vi "VNA_Easy_Loop_Sweep_CenterFreq.vi"(4 "CentreF Start (Hz)":dbl=1000000000.0 format="%#_8p", 5 "Transport":refnum<class "Transport.lvclass">, 7 "VNA Address":refnum<visa-resource-name>="GPIB0::15::INSTR", 9 "sweep type (0 : linear)":u16(ring) items=["linear sweep", "logarithmic sweep", "frequency list", "CW time sweep", "power sweep"], 10 "sweep time (sec)":dbl=1.0 format="%.2f", 11 "num points":u16(ring)=8 items=["3", "11", "21 ('20) / 26 ('53)", "51", "101", "201", "401", "801", "1601"]) -> (2 "Polar plot":cluster{dbl[], sgl[]}[](graph))   [LabVIEW 2020]
uses:
  <userlib>/LevyLab/Transport/Transport/Transport.lvclass
  <userlib>/LevyLab/Transport/Transport/Transport.lvclass/Transport.ctl
  <userlib>/LevyLab/Transport/Control Experiment/Control Experiment.lvclass/Control Experiment.ctl
  <userlib>/LevyLab/Transport/Control Experiment/Control Experiment.lvclass
  <userlib>/LevyLab/Instrument Framework/Instrument Types/Cryostat/Instrument.Cryostat.lvclass
  <instrlib>/Agilent 87XX Series/Agilent 87XX Series.lvlib
panel:
  in  "Power (dBm)":dbl=10.0
  in  "CentreF Step (Hz)":dbl=50000000.0 format="%#_8p"
  in  "CentreF End (Hz)":dbl=1200000000.0 format="%#_8p"
  out "Data 2":cluster{dbl[], dbl[]}[](graph)
  out "B Field (T)":dbl=-0.0001169
  out "Temperature (K)":dbl=300.0009
  in  "Vg (V)":dbl
  in  "Ids (mA)":dbl=9.5
  in  "Vds (V)":dbl=1.3
  in  "Experiment Description":string="D1 1/2\nT = 300K\nVdc1 =AO1 (100kohm shunt) = 0 V\nVcd2 = AO2  (100kohm shunt) = 0 V\nP_vna = 10 dBm \nCentreF = 1G to 1.2G\nSpan=50M"
  in  "Experiment Folder":string="06-100K_bias0V"
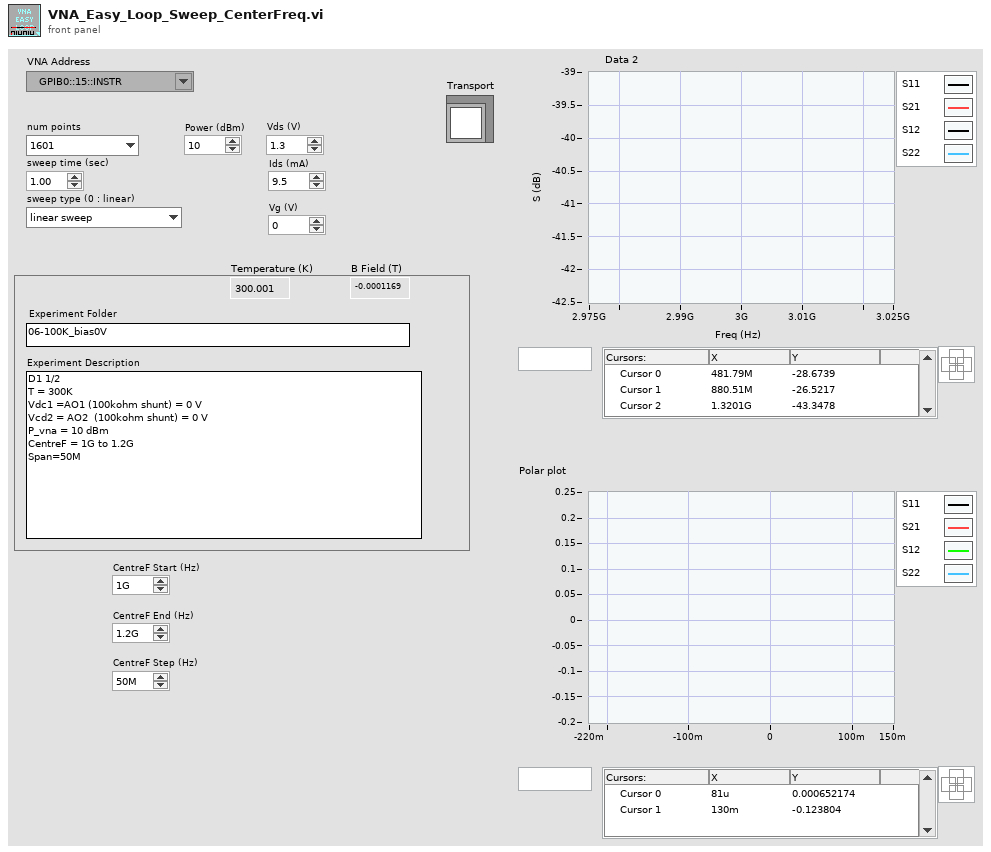
[diagram p1: front panel]
types:
  T1 = enum32{"Bad", "Idle", "Run top level", "Running"}
  T2 = typedef "Control Experiment.lvclass/Instrument Classes--cluster.ctl" = cluster{"DAQ":refnum<class "Instrument.LockinAPI.lvclass">, "Amplifier":refnum<class "Instrument.Amplifier.lvclass">, "Temperature":refnum<class "Instrument.Cryostat.lvclass">, "Magnet":refnum<class "Instrument.Cryostat.lvclass">, "Rotator":refnum<class "Instrument.Cryostat.lvclass">, "Level":refnum<class "Instrument.Cryostat.lvclass">, "Capacitance":refnum<class "Instrument.CBridge.lvclass">, "Delay Line":refnum<class "Instrument.DelayLine.lvclass">, "Strain Cell":refnum<class "Instrument.Strain.lvclass">, "VNA":refnum<class "Instrument.VNA.lvclass">, "Source":refnum<class "Instrument.VSource.lvclass">}
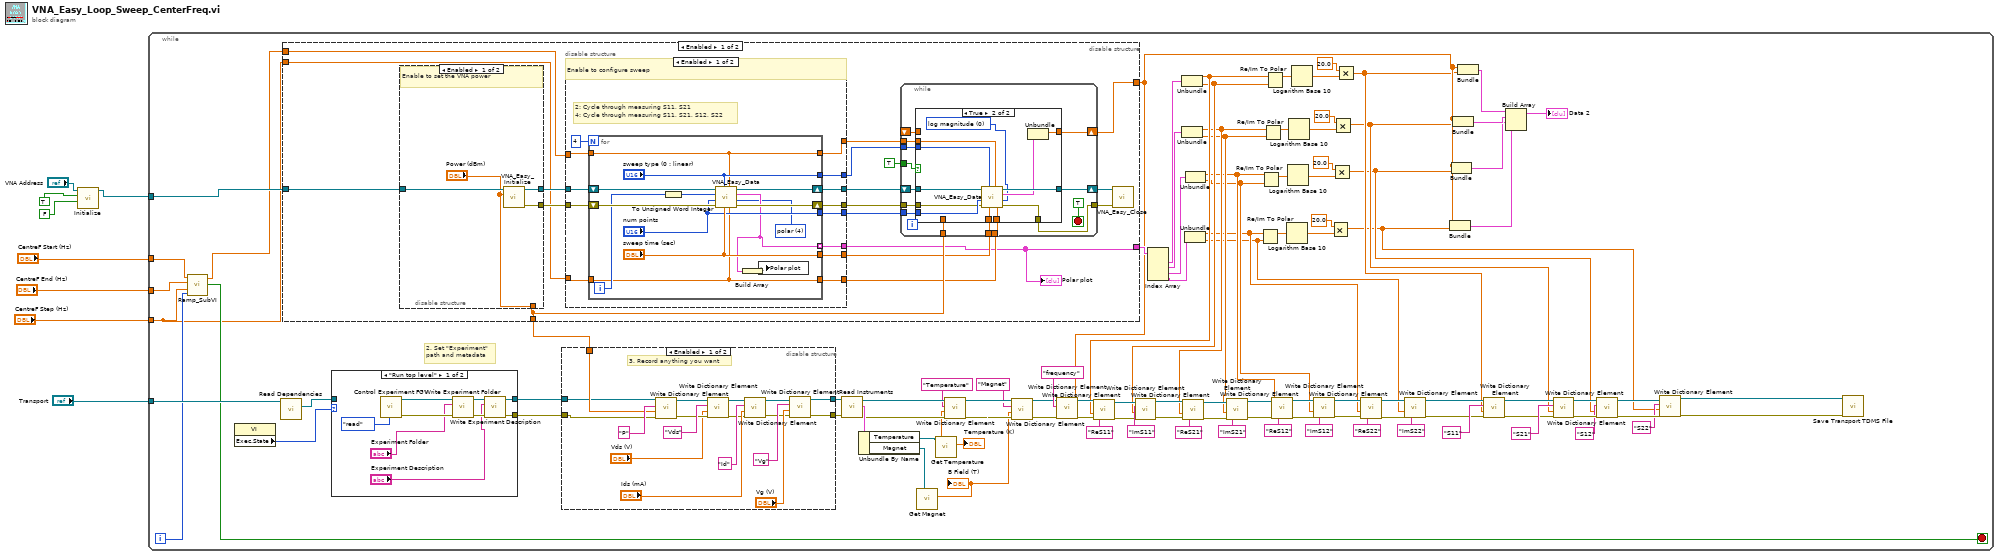
[diagram p0: block diagram]
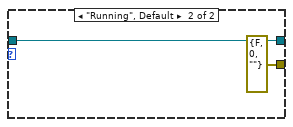
[diagram p2: hidden frame]
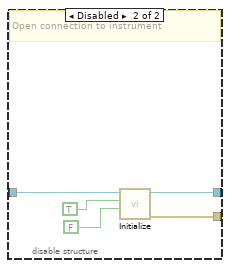
[diagram p5: hidden frame]
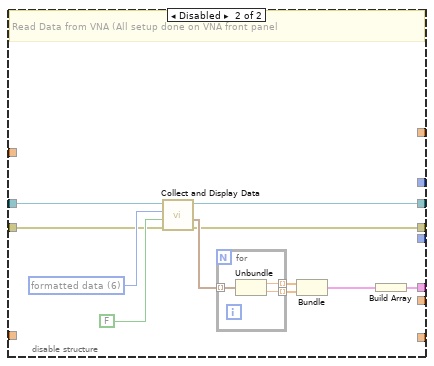
[diagram p6: hidden frame]
diagram:
  n1 = call <instrlib>:"Initialize.vi"("reset"=FALSE, "ID query"=TRUE, "VISA resource name"="VNA Address") -> ("VISA resource name out"=w3:refnum<visa-resource-name>)  [unwired: 7 in, 1 out]
  n2 = while {
    tunnel: "Transport" -> [w74]
    tunnel: "CentreF Start (Hz)" -> [w14]
    tunnel: w3 -> [w15]
    tunnel: "CentreF End (Hz)" -> [w13]
    tunnel: "CentreF Step (Hz)" -> [w9]
    i -> [w12]
    stop <- w11 stop-if-true
    # "2. Set \"Experiment\"\npath and metadata"
    n3 = call <userlib>:"Ramp_SubVI.vi"("index"=w12, "step"=w9, "end"=w13, "start"=w14) -> ("Stop?"=w11:bool, "Numeric"=w10:dbl)  [unwired: 1 in]
    n4 = property class="VI"() -> ("Exec.State"=w77:T1)  [unwired: 2 in, 2 out]
    n5 = call <userlib>:"Read Dependencies.vi"("Transport"=w74) -> ("C.E."=w73:refnum<class "Control Experiment.lvclass">)  [unwired: 8 in, 2 out]
    n6 = disable-structure shown="Enabled" {
      disable-tunnel: [w146 _] -> w72
      disable-tunnel: [w154 _] -> w103
      disable-tunnel: [w155 _] -> w30
      disable-tunnel: w15 -> [w145 _]
      disable-tunnel: w10 -> [w144 _]
      disable-tunnel: w9 -> [w143 _]
      frame Enabled {
        n7 = disable-structure shown="Enabled" {
          disable-tunnel: w145 -> [w192 w195]
          disable-tunnel: [w191 w193] -> w159
          disable-tunnel: [w190 w194] -> w158
          disable-tunnel: ["Power (dBm)" _] -> w154
          frame Enabled {
            # "Enable to set the VNA power"
            n8 = call "VNA_Easy_Initialize.vi"("Power (dbm)"="Power (dBm)", "VISA Refnum in"=w192) -> ("error out"=w190:errorcluster, "VISA Refnum out"=w191:refnum<visa-resource-name>)  [unwired: 8 in]
          }
          frame Disabled {
            # "Open connection to instrument"
            n9 = call <instrlib>:"Initialize.vi"("reset"=FALSE, "ID query"=TRUE, "VISA resource name"=w195) -> ("error out"=w194:errorcluster, "VISA resource name out"=w193:refnum<visa-resource-name>)  [unwired: 7 in]
          }
        }
        n10 = disable-structure shown="Enabled" {
          disable-tunnel: w159 -> [w210 w229]
          disable-tunnel: w158 -> [w209 w230]
          disable-tunnel: [w208 w227] -> w153
          disable-tunnel: [w207 w228] -> w157
          disable-tunnel: [w206 w225] -> w146
          disable-tunnel: [w204 _] -> w151
          disable-tunnel: [w203 _] -> w150
          disable-tunnel: [w202 _] -> w149
          disable-tunnel: [w201 _] -> w148
          disable-tunnel: [w200 _] -> w147
          disable-tunnel: w144 -> [w199 _]
          disable-tunnel: w143 -> [w198 _]
          frame Enabled {
            # "2: Cycle through measuring S11, S21\n4: Cycle through measuring S11, S21, S12, S22"
            # "Enable to configure sweep"
            n11 = for {
              N: 4 -> [_]
              tunnel: [w214] -> w206 mode=indexing
              shift-right: [w221] -> w207
              shift-left: w210 -> [w224]
              shift-right: [w222] -> w208
              shift-left: w209 -> [w223]
              tunnel: ["sweep type (0 : linear)"] -> w204
              tunnel: [w211] -> w203
              tunnel: ["sweep time (sec)"] -> w202
              tunnel: [w212] -> w201
              tunnel: ["num points"] -> w200
              tunnel: w199 -> [w212]
              tunnel: w198 -> [w211]
              i -> [w220]
              w213 = u16 4 items=["log magnitude", "phase", "delay", "Smith chart", "polar", "linear magnitude", "standing wave ratio", "real", "imaginary"] ("format (0 : log mag)")
              n12 = To Unsigned Word Integer(number=w220) -> (unsigned 16bit integer=w219:u16)
              n13 = call "VNA_Easy_Data.vi"("format (0 : log mag)"=w213, "stop/span"=w211, "start/center"=w212, "sweep time (sec)"="sweep time (sec)", "sweep type (0 : linear)"="sweep type (0 : linear)", "error in (no error)"=w223, "num points"="num points", "measurement (0 : S11)"=w219, "VISA Refnum in"=w224) -> ("error out"=w222:errorcluster, "Data"=w214:cluster{dbl[], sgl[]}, "VISA Refnum out"=w221:refnum<visa-resource-name>)
              n14 = Build Array(w214) -> (w215:cluster{dbl[], sgl[]}[])
              n15 = local write "Polar plot"(w215) -> ()
            }
          }
          frame Disabled {
            w235 = u16 6 items=["raw data array 1", "raw data array 2", "raw data array 3", "raw data array 4", "error-corrected data", "error-corrected trace memory", "formatted data", "formatted memory", "formatted data / memory", "formatted data - memory"] ("data type (6 : formatted data)")
            # "Read Data from VNA (All setup done on VNA front panel"
            n16 = call <instrlib>:"Collect and Display Data.vi"("error in (no error)"=w230, "save to file"=FALSE, "data type (6 : formatted data)"=w235, "VISA resource name"=w229) -> ("error out"=w227:errorcluster, "data values"=w232:cluster{"real / stim":dbl, "imag / resp":sgl}[], "VISA resource name out"=w228:refnum<visa-resource-name>)  [unwired: 4 in, 1 out]
            n17 = for {
              tunnel: w232 -> [w238] mode=indexing
              tunnel: [w237] -> w233 mode=indexing
              tunnel: [w236] -> w234 mode=indexing
              n18 = Unbundle(w238) -> ("real / stim"=w237:dbl, "imag / resp"=w236:sgl)
            }
            n19 = Bundle(w233, w234) -> (w226:cluster{dbl[], sgl[]})  [unwired: 1 in]
            n20 = Build Array(w226) -> (w225:cluster{dbl[], sgl[]}[])
          }
        }
        "Polar plot" <- w146
        n21 = while {
          shift-right: [w172] -> w156
          shift-left: w157 -> [w173]
          shift-right: [w170] -> w155
          shift-left: _ -> [w169]
          tunnel: TRUE ("First Call?: T/F") -> [w168]
          tunnel: w154 -> [w167]
          tunnel: w153 -> [w166]
          tunnel: [w165] -> w152
          tunnel: w151 -> [w164]
          tunnel: w150 -> [w163]
          tunnel: w149 -> [w162]
          tunnel: w148 -> [w161]
          tunnel: w147 -> [w160]
          stop <- TRUE stop-if-true
          n22 = case shown="True" w168 {
            tunnel: w173 -> [w175 w178]
            tunnel: [w175 w188] -> w172
            tunnel: [w176 w186] -> w170
            tunnel: w169 -> [w176 _]
            tunnel: w167 -> [_ _]
            tunnel: w166 -> [w174 w177]
            tunnel: [w174 w185] -> w165
            tunnel: w164 -> [_ w184]
            tunnel: w163 -> [_ w183]
            tunnel: w162 -> [_ w182]
            tunnel: w161 -> [_ w181]
            tunnel: w160 -> [_ w180]
            frame False {
            }
            frame True {
              w179 = u16 0 items=["log magnitude", "phase", "delay", "Smith chart", "polar", "linear magnitude", "standing wave ratio", "real", "imaginary"] ("format (0 : log mag)")
              n23 = call "VNA_Easy_Data.vi"("format (0 : log mag)"=w179, "stop/span"=w183, "start/center"=w181, "sweep time (sec)"=w182, "sweep type (0 : linear)"=w184, "error in (no error)"=w177, "num points"=w180, "VISA Refnum in"=w178) -> ("error out"=w185:errorcluster, "Data"=w187:cluster{dbl[], sgl[]}, "VISA Refnum out"=w188:refnum<visa-resource-name>)  [unwired: 1 in]
              n24 = Unbundle(w187) -> (w186:dbl[])  [unwired: 1 out]
            }
          }
        }
        n25 = call "VNA_Easy_Close.vi"("error in (no error)"=w152, "VISA Refnum in"=w156) -> ()  [unwired: 9 in, 1 out]
      }
      frame Disabled {
      }
    }
    n26 = case shown="\"Run top level\"" w77 {
      tunnel: [w115 errorcluster {"status"=FALSE, "code"=0, "source"=""} ("error out")] -> w75
      tunnel: [w114 w121] -> w76
      tunnel: w73 -> [_ w121]
      frame "Run top level" {
        n27 = call <userlib>:"Control Experiment FGV.vi"("Function"=enum16{"read", "write"}."read") -> ("error out"=w118:errorcluster, "Control Experiment.lvclass out"=w119:refnum<class "Control Experiment.lvclass">)  [unwired: 9 in]
        n28 = call <userlib>:"Write Experiment Folder.vi"("error in (no error)"=w118, "Experiment Folder"="Experiment Folder", "Control Experiment in"=w119) -> ("error out"=w116:errorcluster, "Control Experiment out"=w117:refnum<class "Control Experiment.lvclass">)  [unwired: 7 in]
        n29 = call <userlib>:"Write Experiment Description.vi"("error in (no error)"=w116, "Experiment Description"="Experiment Description", "Control Experiment in"=w117) -> ("error out"=w115:errorcluster, "Control Experiment out"=w114:refnum<class "Control Experiment.lvclass">)  [unwired: 7 in]
      }
      frame "Running", Default {
      }
    }
    n30 = disable-structure shown="Enabled" {
      disable-tunnel: w76 -> [w131 w141]
      disable-tunnel: w75 -> [w130 w140]
      disable-tunnel: [w136 w141] -> w102
      disable-tunnel: [w122 w140] -> w101
      disable-tunnel: w103 -> [w132 _]
      frame Enabled {
        # "3. Record anything you want"
        n31 = call <userlib>:"Write Dictionary Element.vi"("error in (no error)"=w130, "value"=w132, "key"="P", "Control Experiment in"=w131) -> ("error out"=w128:errorcluster, "Control Experiment out"=w129:refnum<class "Control Experiment.lvclass">)  [unwired: 6 in]
        n32 = call <userlib>:"Write Dictionary Element.vi"("error in (no error)"=w128, "value"="Vds (V)", "key"="Vds", "Control Experiment in"=w129) -> ("error out"=w125:errorcluster, "Control Experiment out"=w138:refnum<class "Control Experiment.lvclass">)  [unwired: 6 in]
        n33 = call <userlib>:"Write Dictionary Element.vi"("error in (no error)"=w125, "value"="Ids (mA)", "key"="Id", "Control Experiment in"=w138) -> ("error out"=w123:errorcluster, "Control Experiment out"=w137:refnum<class "Control Experiment.lvclass">)  [unwired: 6 in]
        n34 = call <userlib>:"Write Dictionary Element.vi"("error in (no error)"=w123, "value"="Vg (V)", "key"="Vg", "Control Experiment in"=w137) -> ("error out"=w122:errorcluster, "Control Experiment out"=w136:refnum<class "Control Experiment.lvclass">)  [unwired: 6 in]
      }
      frame Disabled {
      }
    }
    n35 = call <userlib>:"Read Instruments.vi"("error in (no error)"=w101, "Control Experiment in"=w102) -> ("error out"=w97:errorcluster, "Instruments"=w100:T2, "Control Experiment out"=w96:refnum<class "Control Experiment.lvclass">)  [unwired: 7 in]
    n36 = Unbundle By Name(w100) -> ("Temperature"=w98:refnum<class "Instrument.Cryostat.lvclass">, "Magnet"=w99:refnum<class "Instrument.Cryostat.lvclass">)
    n37 = call-dynamic "Get Magnet.vi"("Instrument.Cryostat in"=w99) -> ("B Field (T)"=w88:dbl)  [unwired: 6 in, 4 out]
    "B Field (T)" <- w88
    n38 = call-dynamic "Get Temperature.vi"("Instrument.Cryostat in"=w98) -> ("Temperature (K)"=w95:dbl)  [unwired: 6 in, 4 out]
    "Temperature (K)" <- w95
    n39 = call <userlib>:"Write Dictionary Element.vi"("error in (no error)"=w97, "value"=w95, "key"="Temperature", "Control Experiment in"=w96) -> ("error out"=w90:errorcluster, "Control Experiment out"=w93:refnum<class "Control Experiment.lvclass">)  [unwired: 6 in]
    n40 = call <userlib>:"Write Dictionary Element.vi"("error in (no error)"=w90, "value"=w88, "key"="Magnet", "Control Experiment in"=w93) -> ("error out"=w91:errorcluster, "Control Experiment out"=w92:refnum<class "Control Experiment.lvclass">)  [unwired: 6 in]
    n41 = call <userlib>:"Write Dictionary Element.vi"("error in (no error)"=w91, "value"=w30, "key"="frequency", "Control Experiment in"=w92) -> ("error out"=w62:errorcluster, "Control Experiment out"=w64:refnum<class "Control Experiment.lvclass">)  [unwired: 6 in]
    n42 = Index Array(array=w72) -> (element #1=w110:cluster{dbl[], sgl[]}, element #2=w104:cluster{dbl[], sgl[]}, element #3=w80:cluster{dbl[], sgl[]}, element #4=w78:cluster{dbl[], sgl[]})  [unwired: 4 in]
    n43 = Unbundle(w110) -> (w40:dbl[], w39:sgl[])
    n44 = call <userlib>:"Write Dictionary Element.vi"("error in (no error)"=w62, "value"=w40, "key"="ReS11", "Control Experiment in"=w64) -> ("error out"=w61:errorcluster, "Control Experiment out"=w63:refnum<class "Control Experiment.lvclass">)  [unwired: 6 in]
    n45 = call <userlib>:"Write Dictionary Element.vi"("error in (no error)"=w61, "value"=w39, "key"="ImS11", "Control Experiment in"=w63) -> ("error out"=w56:errorcluster, "Control Experiment out"=w58:refnum<class "Control Experiment.lvclass">)  [unwired: 6 in]
    n46 = Unbundle(w104) -> (w26:dbl[], w25:sgl[])
    n47 = call <userlib>:"Write Dictionary Element.vi"("error in (no error)"=w56, "value"=w26, "key"="ReS21", "Control Experiment in"=w58) -> ("error out"=w55:errorcluster, "Control Experiment out"=w57:refnum<class "Control Experiment.lvclass">)  [unwired: 6 in]
    n48 = Unbundle(w78) -> (w22:dbl[], w21:sgl[])
    n49 = Unbundle(w80) -> (w24:dbl[], w23:sgl[])
    n50 = call <userlib>:"Write Dictionary Element.vi"("error in (no error)"=w55, "value"=w25, "key"="ImS21", "Control Experiment in"=w57) -> ("error out"=w43:errorcluster, "Control Experiment out"=w44:refnum<class "Control Experiment.lvclass">)  [unwired: 6 in]
    n51 = Re/Im To Polar(2:w21, 3:w22) -> (1:w32:dbl[])  [unwired: 1 out]
    n52 = Re/Im To Polar(2:w23, 3:w24) -> (1:w35:dbl[])  [unwired: 1 out]
    n53 = Re/Im To Polar(2:w25, 3:w26) -> (1:w16:dbl[])  [unwired: 1 out]
    n54 = Re/Im To Polar(2:w39, 3:w40) -> (1:w68:dbl[])  [unwired: 1 out]
    n55 = call <userlib>:"Write Dictionary Element.vi"("error in (no error)"=w43, "value"=w24, "key"="ReS12", "Control Experiment in"=w44) -> ("error out"=w51:errorcluster, "Control Experiment out"=w52:refnum<class "Control Experiment.lvclass">)  [unwired: 6 in]
    n56 = Logarithm Base 10(1:w32) -> (0:w31:dbl[])
    n57 = Logarithm Base 10(1:w35) -> (0:w34:dbl[])
    n58 = Logarithm Base 10(1:w16) -> (0:w37:dbl[])
    n59 = Logarithm Base 10(1:w68) -> (0:w67:dbl[])
    n60 = call <userlib>:"Write Dictionary Element.vi"("error in (no error)"=w51, "value"=w23, "key"="ImS12", "Control Experiment in"=w52) -> ("error out"=w46:errorcluster, "Control Experiment out"=w48:refnum<class "Control Experiment.lvclass">)  [unwired: 6 in]
    n61 = Multiply(x=20.0, y=w31) -> (x*y=w17:dbl[])
    n62 = Multiply(x=20.0, y=w34) -> (x*y=w18:dbl[])
    n63 = Multiply(x=20.0, y=w37) -> (x*y=w19:dbl[])
    n64 = Multiply(x=20.0, y=w67) -> (x*y=w20:dbl[])
    n65 = call <userlib>:"Write Dictionary Element.vi"("error in (no error)"=w46, "value"=w22, "key"="ReS22", "Control Experiment in"=w48) -> ("error out"=w45:errorcluster, "Control Experiment out"=w47:refnum<class "Control Experiment.lvclass">)  [unwired: 6 in]
    n66 = call <userlib>:"Write Dictionary Element.vi"("error in (no error)"=w45, "value"=w21, "key"="ImS22", "Control Experiment in"=w47) -> ("error out"=w41:errorcluster, "Control Experiment out"=w42:refnum<class "Control Experiment.lvclass">)  [unwired: 6 in]
    n67 = Bundle(w30, w17) -> (w27:cluster{dbl[], dbl[]})  [unwired: 1 in]
    n68 = Bundle(w30, w18) -> (w28:cluster{dbl[], dbl[]})  [unwired: 1 in]
    n69 = Bundle(w30, w19) -> (w29:cluster{dbl[], dbl[]})  [unwired: 1 in]
    n70 = Bundle(w30, w20) -> (w71:cluster{dbl[], dbl[]})  [unwired: 1 in]
    n71 = call <userlib>:"Write Dictionary Element.vi"("error in (no error)"=w41, "value"=w20, "key"="S11", "Control Experiment in"=w42) -> ("error out"=w106:errorcluster, "Control Experiment out"=w105:refnum<class "Control Experiment.lvclass">)  [unwired: 6 in]
    n72 = Build Array(w71, w29, w28, w27) -> (→"Data 2":cluster{dbl[], dbl[]}[])
    n73 = call <userlib>:"Write Dictionary Element.vi"("error in (no error)"=w106, "value"=w19, "key"="S21", "Control Experiment in"=w105) -> ("error out"=w84:errorcluster, "Control Experiment out"=w87:refnum<class "Control Experiment.lvclass">)  [unwired: 6 in]
    n74 = call <userlib>:"Write Dictionary Element.vi"("error in (no error)"=w84, "value"=w18, "key"="S12", "Control Experiment in"=w87) -> ("error out"=w83:errorcluster, "Control Experiment out"=w86:refnum<class "Control Experiment.lvclass">)  [unwired: 6 in]
    n75 = call <userlib>:"Write Dictionary Element.vi"("error in (no error)"=w83, "value"=w17, "key"="S22", "Control Experiment in"=w86) -> ("error out"=w79:errorcluster, "Control Experiment out"=w85:refnum<class "Control Experiment.lvclass">)  [unwired: 6 in]
    n76 = call <userlib>:"Save Transport TDMS File.vi"("error in (no error)"=w79, "Control Experiment in"=w85) -> ()  [unwired: 8 in, 2 out]
  }
